vi "GetText.vi"(8 "error in":errorcluster, 11 "SwitchACIR Channel in":refnum<class "SwitchACIR Channel.lvclass">) -> (0 "error out":errorcluster, 1 "additional text":string, 2 "text":string, 3 "SwitchACIR Channel out":refnum<class "SwitchACIR Channel.lvclass">, 4 "glyph":string)   [LabVIEW 2025, in "SwitchACIR Channel.lvclass"]
doc: "Copyright 2017 National Instruments Corporation\n\nLicensed under the Apache License, Version 2.0 (the \"License\"); you may not use this file except in compliance with the License. You may obtain a copy of the License at http://www.apache.org/licenses/LICENSE-2.0\nUnless required by applicable law or agreed to in writing, software distributed under the License is distributed on an \"AS IS\" BASIS, WITHOUT WARRANTIES OR CONDITIONS OF ANY KIND, either express or implied. See the License for the specific language governing permissions and limitations under the License."
uses:
  SwitchACIR Channel.lvclass
  SwitchACIR Channel.lvclass/SwitchACIR Channel.ctl
  SwitchACIR Channel configuration/SwitchACIR Channel configuration.lvclass
  C:/Users/Public/Documents/Sandia National Labs/TSS Plugin/Abstract Engine.lvlibp/Channel configuration/Channel configuration.lvclass
  Users/Public/Documents/Sandia National Labs/TSS Plugin/Abstract Engine.lvlibp/Channel configuration/Read Channel Setting.vi
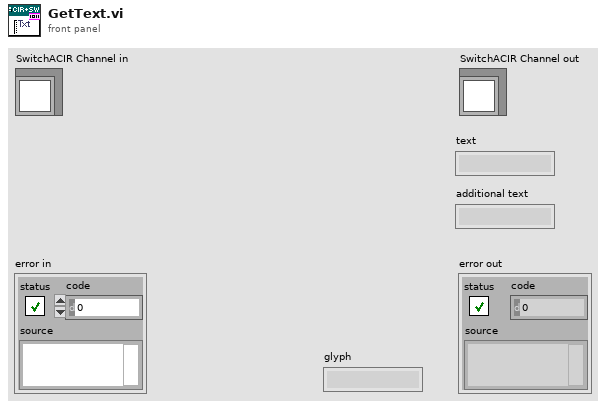
[diagram p1: front panel]
types:
  T1 = typedef "Abstract Engine.lvlibp/Channel configuration.lvclass/Default Channel.ctl" = cluster{"Address":string, "SW Alias":string, "Enabled":bool, "Type":string, "Description":string}
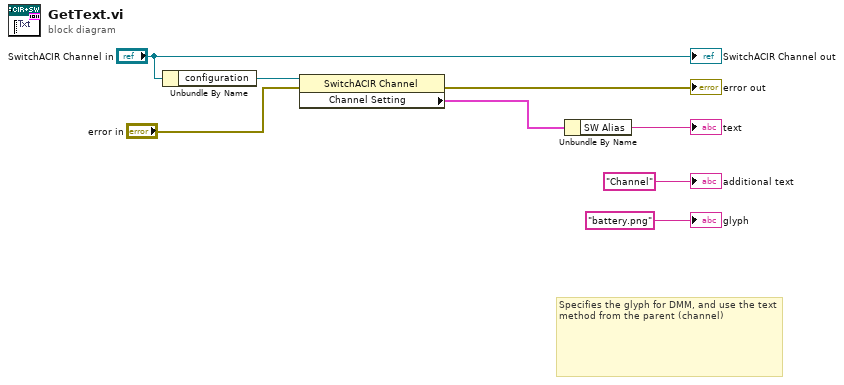
[diagram p0: block diagram]
diagram:
  # "Specifies the glyph for DMM, and use the text method from the parent (channel)"
  n1 = Unbundle By Name("SwitchACIR Channel in") -> ("configuration"=w4:refnum<class "SwitchACIR Channel configuration.lvclass">)
  n2 = property class="SwitchACIR Channel"(reference=w4, error in="error in") -> (error out=→"error out":errorcluster, "Channel Setting"=w2:T1)  [unwired: 1 out]
  n3 = Unbundle By Name(w2) -> ("SW Alias"=→"text":string)
  "SwitchACIR Channel out" <- "SwitchACIR Channel in"
  "additional text" <- "Channel" ("additional text")
  "glyph" <- "battery.png" ("glyph")
